vi "Target Generate Metadata v2.vi"() -> (0 "Data":dbl[](array[numeric]), 3 "channel name(s)":string[](array[string]))   [LabVIEW 2018]
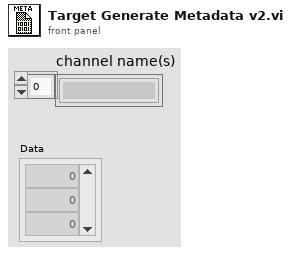
[diagram p1: front panel]
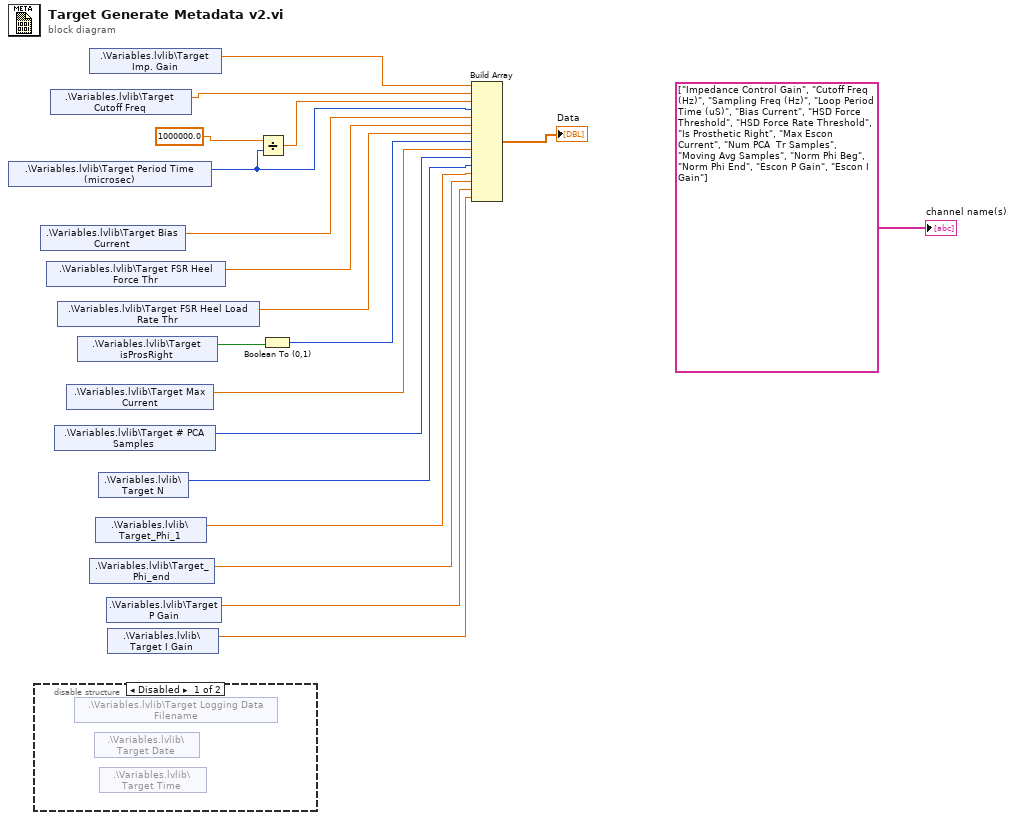
[diagram p0: block diagram]
diagram:
  n1 = shared-variable ".\\Variables.lvlib\\Target Period Time (microsec)"() -> (w8:u16)  [unwired: 1 in, 1 out]
  n2 = disable-structure shown="Disabled" {
    frame Disabled {
      n3 = shared-variable ".\\Variables.lvlib\\Target Logging Data Filename"() -> ()  [unwired: 1 in, 2 out]
      n4 = shared-variable ".\\Variables.lvlib\\Target Date"() -> ()  [unwired: 1 in, 2 out]
      n5 = shared-variable ".\\Variables.lvlib\\Target Time"() -> ()  [unwired: 1 in, 2 out]
    }
    frame Enabled {
    }
  }
  n6 = shared-variable ".\\Variables.lvlib\\Target Bias Current"() -> (w13:dbl)  [unwired: 1 in, 1 out]
  n7 = shared-variable ".\\Variables.lvlib\\Target FSR Heel Force Thr"() -> (w12:dbl)  [unwired: 1 in, 1 out]
  n8 = shared-variable ".\\Variables.lvlib\\Target Cutoff Freq"() -> (w15:dbl)  [unwired: 1 in, 1 out]
  n9 = shared-variable ".\\Variables.lvlib\\Target # PCA Samples"() -> (w6:u16)  [unwired: 1 in, 1 out]
  n10 = shared-variable ".\\Variables.lvlib\\Target FSR Heel Load Rate Thr"() -> (w11:dbl)  [unwired: 1 in, 1 out]
  n11 = shared-variable ".\\Variables.lvlib\\Target Max Current"() -> (w7:dbl)  [unwired: 1 in, 1 out]
  n12 = shared-variable ".\\Variables.lvlib\\Target isProsRight"() -> (w10:bool)  [unwired: 1 in, 1 out]
  n13 = shared-variable ".\\Variables.lvlib\\Target Imp. Gain"() -> (w17:dbl)  [unwired: 1 in, 1 out]
  n14 = shared-variable ".\\Variables.lvlib\\Target_Phi_end"() -> (w3:dbl)  [unwired: 1 in, 1 out]
  n15 = shared-variable ".\\Variables.lvlib\\Target_Phi_1"() -> (w4:dbl)  [unwired: 1 in, 1 out]
  n16 = shared-variable ".\\Variables.lvlib\\Target N"() -> (w5:u32)  [unwired: 1 in, 1 out]
  n17 = shared-variable ".\\Variables.lvlib\\Target P Gain"() -> (w2:dbl)  [unwired: 1 in, 1 out]
  n18 = shared-variable ".\\Variables.lvlib\\Target I Gain"() -> (w1:dbl)  [unwired: 1 in, 1 out]
  n19 = Divide(x=1000000.0, y=w8) -> (x/y=w14:dbl)
  n20 = Boolean To (0,1)(Boolean=w10) -> (0, 1=w9:i16)
  n21 = Build Array "Build Array"(w17, w15, w14, w8, w13, w12, w11, w9, w7, w6, w5, w4, w3, w2, w1) -> (→"Data":dbl[])
  "channel name(s)" <- string[] ["Impedance Control Gain", "Cutoff Freq (Hz)", "Sampling Freq (Hz)", "Loop Period Time (uS)", "Bias Current", "HSD Force Threshold", "HSD Force Rate Threshold", "Is Prosthetic Right", "Max Escon Current", "Num PCA  Tr Samples", "Moving Avg Samples", "Norm Phi Beg", "Norm Phi End", "Escon P Gain", "Escon I Gain"]
